vi "Parse Array.vi"(0 "JSON String":string, 5 "Index In":i32, 11 "error in (no error)":errorcluster) -> (4 "Variant out":variant, 6 "Index Out":i32, 15 "error out":errorcluster)   [LabVIEW 2020, in "Variant JSON API.lvlib"]
uses:
  Variant JSON API.lvlib
  Errors.ctl
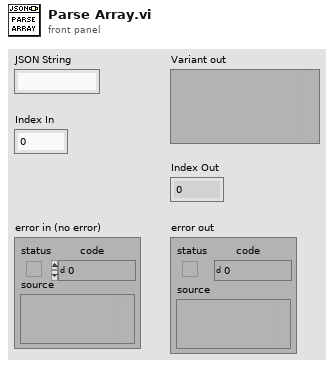
[diagram p1: front panel]
types:
  T1 = typedef "Variant JSON API.lvlib/Errors.ctl" = enum16{"No key", "Key path type", "Array OOB", "Type Mismatch", "Invalid Token", "Invalid Value"}
  T2 = typedef "Variant JSON API.lvlib/Token Type.ctl" = enum16{"NONE", "CURLY_OPEN", "CURLY_CLOSE", "SQUARED_OPEN", "SQUARED_CLOSE", "COLON", "COMMA", "STRING", "NUMBER", "TRUE", "FALSE", "NULL"}
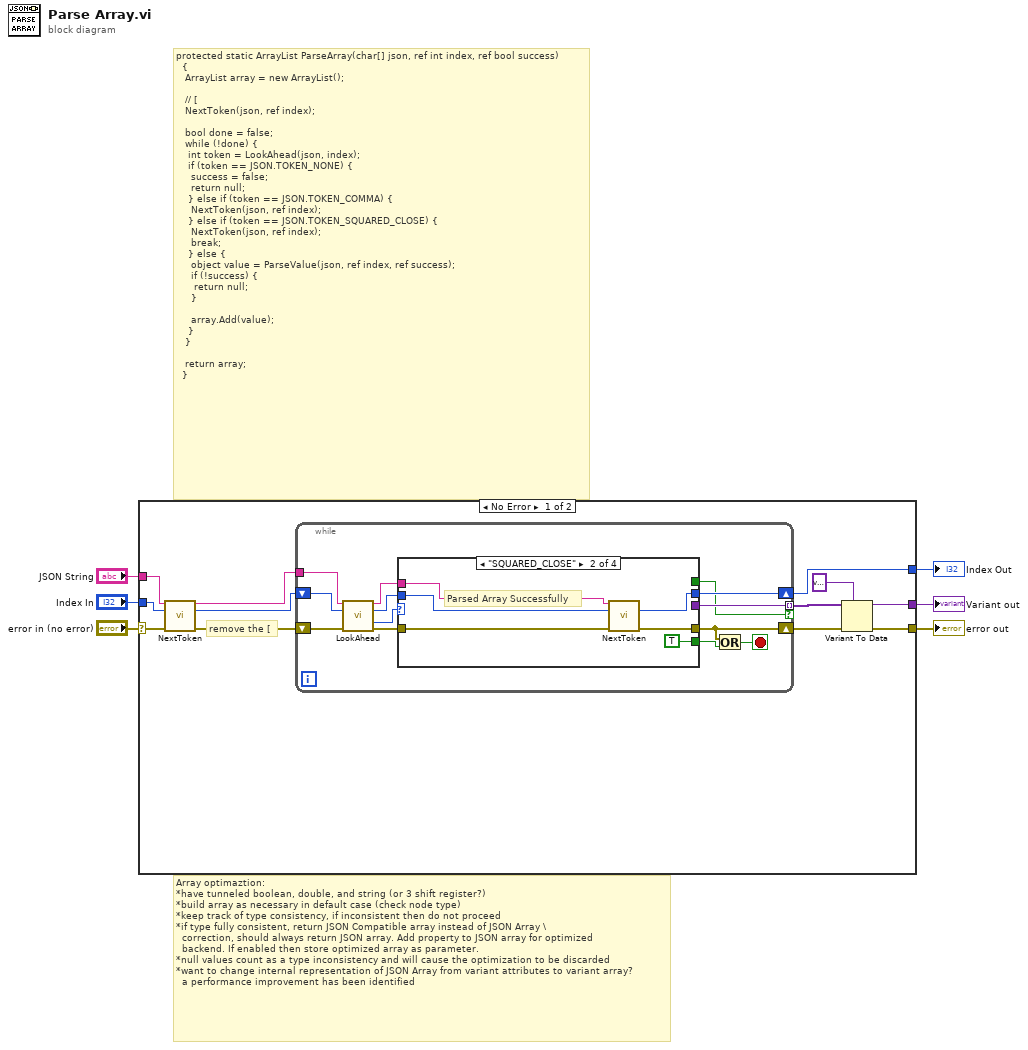
[diagram p0: block diagram]
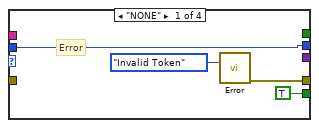
[diagram p2: hidden frame]
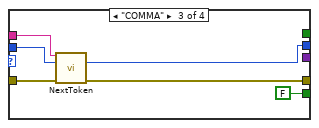
[diagram p3: hidden frame]
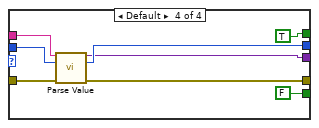
[diagram p4: hidden frame]
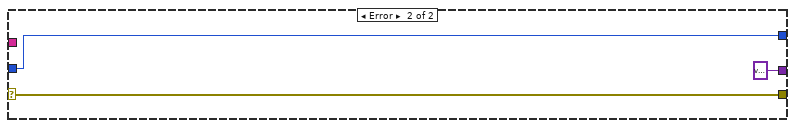
[diagram p5: hidden frame]
diagram:
  # "Array optimaztion:\n*have tunneled boolean, double, and string (or 3 shift register?)\n*build array as necessary in default case (check node type)\n*keep track of type consistency, if inconsistent then do not proceed\n*if type fully consistent, return JSON Compatible array instead of JSON Array \\\n  correction, should always return JSON array. Add property to JSON array for optimized\n  backend. If enabled then store optimized array as parameter.\n*null values count as a type inconsistency and will cause the optimization to be discarded\n*want to change internal representation of JSON Array from variant attributes to variant array?\n  a performance improvement has been identified"
  # "protected static ArrayList ParseArray(char[] json, ref int index, ref bool success)\n\t\t{\n\t\t\tArrayList array = new ArrayList();\n\n\t\t\t// [\n\t\t\tNextToken(json, ref index);\n\n\t\t\tbool done = false;\n\t\t\twhile (!done) {\n\t\t\t\tint token = LookAhead(json, index);\n\t\t\t\tif (token == JSON.TOKEN_NONE) {\n\t\t\t\t\tsuccess = false;\n\t\t\t\t\treturn null;\n\t\t\t\t} else if (token == JSON.TOKEN_COMMA) {\n\t\t\t\t\tNextToken(json, ref index);\n\t\t\t\t} else if (token == JSON.TOKEN_SQUARED_CLOSE) {\n\t\t\t\t\tNextToken(json, ref index);\n\t\t\t\t\tbreak;\n\t\t\t\t} else {\n\t\t\t\t\tobject value = ParseValue(json, ref index, ref success);\n\t\t\t\t\tif (!success) {\n\t\t\t\t\t\treturn null;\n\t\t\t\t\t}\n\n\t\t\t\t\tarray.Add(value);\n\t\t\t\t}\n\t\t\t}\n\n\t\t\treturn array;\n\t\t}"
  n1 = case shown="No Error" "error in (no error)" {
    selector: "error in (no error)" -> [w18 w57]
    tunnel: [w9 w57] -> w5
    tunnel: "Index In" -> [w17 w58]
    tunnel: [w13 w58] -> w3
    tunnel: [w11 variant] -> w1
    tunnel: "JSON String" -> [w12 _]
    frame No Error {
      # "remove the ["
      n2 = call "NextToken.vi"("JSON String"=w12, "Index In"=w17, "error in (no error)"=w18) -> ("JSON String Passthrough"=w15:string, "Index Out"=w16:i32, "error out"=w14:errorcluster)  [unwired: 9 in, 1 out]
      n3 = while {
        shift-right: [w24] -> w13
        shift-left: w16 -> [w30]
        tunnel: w15 -> [w29]
        shift-right: [w21] -> w10
        shift-left: w14 -> [w31]
        tunnel: [w20] -> w8 mode=indexing if=w19
        stop <- w22 stop-if-true
        n4 = call "LookAhead.vi"("JSON String"=w29, "Index"=w30, "error in (no error)"=w31) -> ("JSON String Passthrough"=w25:string, "Index Passthrough"=w26:i32, "TOKEN"=w28:T2, "error out"=w27:errorcluster)  [unwired: 9 in]
        n5 = case shown="\"SQUARED_CLOSE\"" w28 {
          tunnel: w27 -> [_ w41 w45 w55]
          tunnel: [TRUE TRUE FALSE FALSE] -> w23
          tunnel: w26 -> [w34 w40 w46 w54]
          tunnel: w25 -> [_ w39 w47 w53]
          tunnel: [w34 w37 w43 w52] -> w24
          tunnel: [w33 w38 w44 w50] -> w21
          tunnel: [_ _ _ w49] -> w20
          tunnel: [_ _ _ TRUE] -> w19
          frame "NONE" {
            # "Error"
            n6 = call "Error.vi"(5:Errors."Invalid Token") -> ("error out"=w33:errorcluster)  [unwired: 14 in]
          }
          frame "SQUARED_CLOSE" {
            # "Parsed Array Successfully"
            n7 = call "NextToken.vi"("JSON String"=w39, "Index In"=w40, "error in (no error)"=w41) -> ("Index Out"=w37:i32, "error out"=w38:errorcluster)  [unwired: 9 in, 2 out]
          }
          frame "COMMA" {
            n8 = call "NextToken.vi"("JSON String"=w47, "Index In"=w46, "error in (no error)"=w45) -> ("Index Out"=w43:i32, "error out"=w44:errorcluster)  [unwired: 9 in, 2 out]
          }
          frame Default {
            n9 = call "Parse Value.vi"("JSON String"=w53, "Index In"=w54, "error in (no error)"=w55) -> ("Variant out"=w49:variant, "Index Out"=w52:i32, "error out"=w50:errorcluster)  [unwired: 10 in]
          }
        }
        n10 = Or(x=w21, y=w23) -> (x .or. y?=w22:bool)
      }
      n11 = Variant To Data(error in=w10, type=variant, Variant=w8) -> (data=w11:variant, error out=w9:errorcluster)
    }
    frame Error {
    }
  }
  "error out" <- w5
  "Index Out" <- w3
  "Variant out" <- w1
